vi "Apply.vi"(8 "error in":errorcluster, 11 "PCAN-USB Base Strategy in":refnum<class "PCAN-USB Base Strategy.lvclass">) -> (0 "error out":errorcluster, 3 "PCAN-USB Base Strategy out":refnum<class "PCAN-USB Base Strategy.lvclass">)   [LabVIEW 2024, in "PCAN-USB Base Strategy.lvclass"]
uses:
  PCAN-USB Base Strategy.lvclass
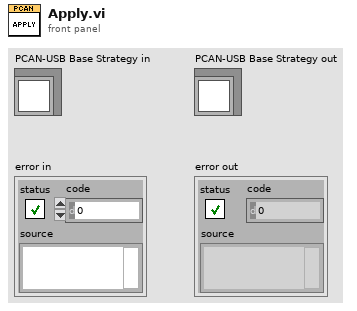
[diagram p1: front panel]
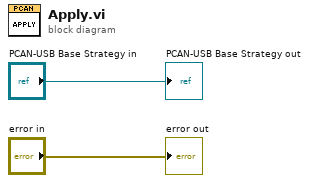
[diagram p0: block diagram]
diagram:
  "error out" <- "error in"
  "PCAN-USB Base Strategy out" <- "PCAN-USB Base Strategy in"
